vi "test_CCDOpenAndClose.vi"(7 "Test should pass":bool=TRUE, 8 "error in":errorcluster, 9 "tear down connection":bool=TRUE, 10 "set-up a connection":bool=TRUE, 11 "device selection":enum16{"monochromator", "CCD", "SCD"}(ring)=enum."CCD") -> (0 "error out":errorcluster)   [LabVIEW 2023]
uses:
  Classes/CCD/CCD.lvclass
  <vilib>/addons/_JKI Toolkits/Caraya/classes/Assert/Assert Equal Value and Type_Variant.vi
  <vilib>/addons/_JKI Toolkits/Caraya/classes/Assert/Assert Not Error.vi
  <vilib>/addons/_JKI Toolkits/Caraya/classes/Test/Test.lvclass
  <vilib>/addons/_JKI Toolkits/Caraya/classes/Assert/Assert.lvclass
panel:
  # "Connector Pane"
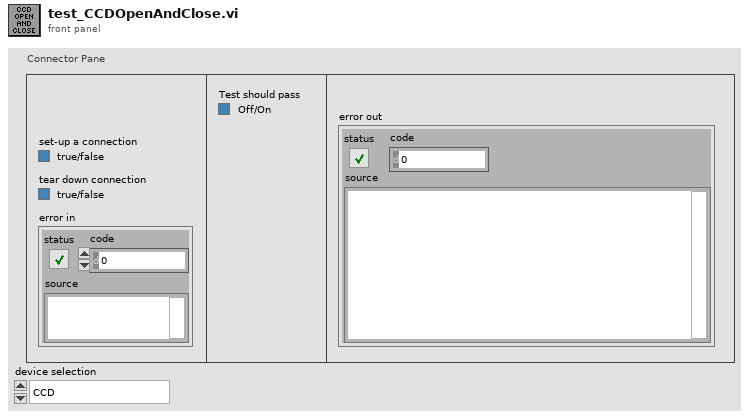
[diagram p1: front panel]
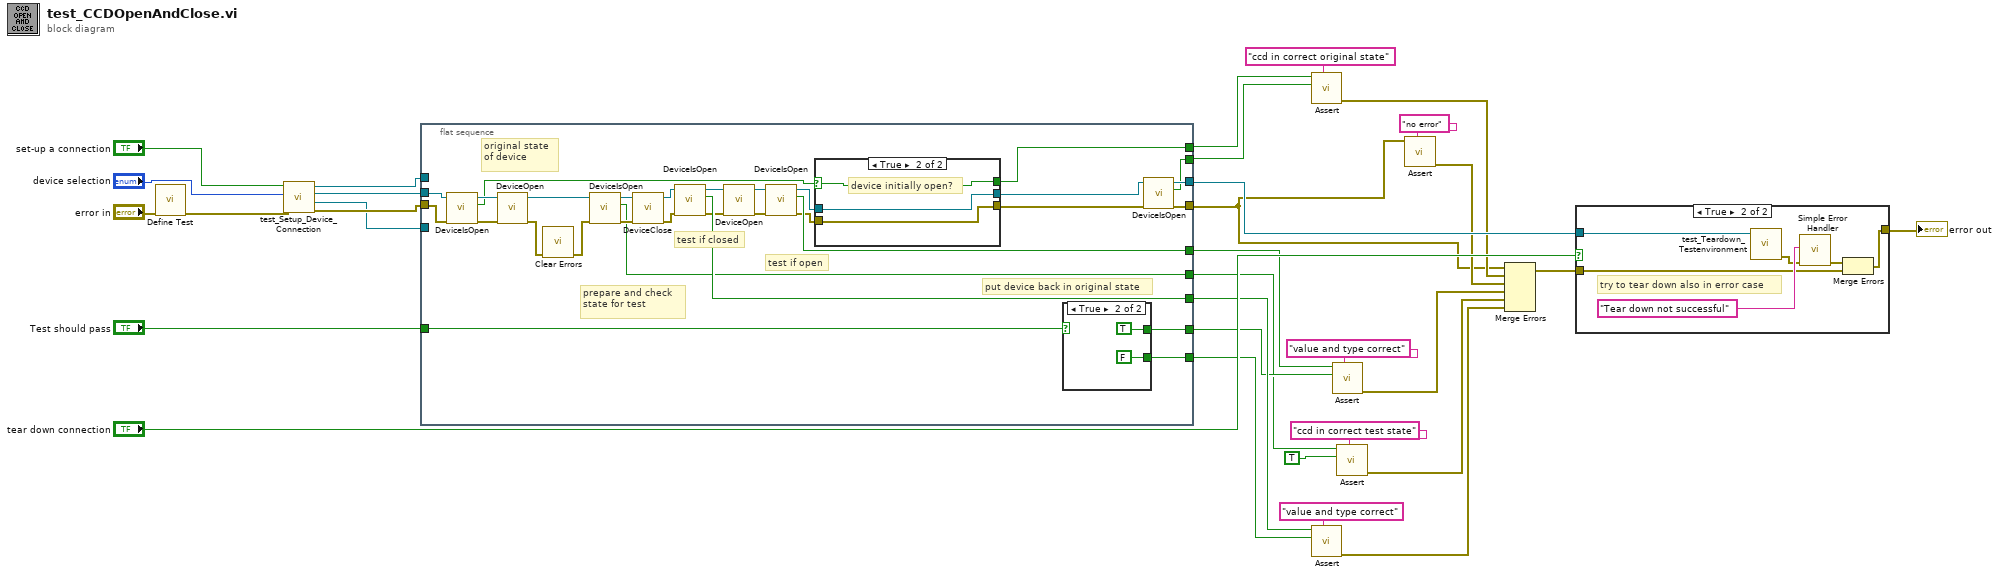
[diagram p0: block diagram]
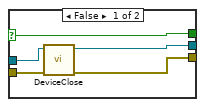
[diagram p2: hidden frame]
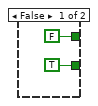
[diagram p3: hidden frame]
diagram:
  n1 = call <vilib>:"Define Test.vi"("error in (no error)"="error in") -> ("error out"=w26:errorcluster)  [unwired: 9 in, 1 out]
  n2 = call "test_Setup_Device_Connection.vi"("error in (no error)"=w26, "device selection"="device selection", "set-up a connection"="set-up a connection") -> ("error out"=w28:errorcluster, "Monochromator out"=w25:refnum<class "Monochromator.lvclass">, "CCD out"=w24:refnum<class "CCD.lvclass">, "SCD out"=w8:refnum<class "SCD.lvclass">)  [unwired: 5 in]
  n3 = flat-sequence {
    tunnel: w28 -> [w61]
    tunnel: w25 -> [_]
    tunnel: w24 -> [w60]
    tunnel: [w36] -> w2
    tunnel: "Test should pass" -> [w62]
    tunnel: [w40] -> w20
    tunnel: [w53] -> w19
    tunnel: [w52] -> w18
    tunnel: [w51] -> w17
    tunnel: [w50] -> w16
    tunnel: [w49] -> w14
    tunnel: [w42] -> w11
    tunnel: [w39] -> w10
    tunnel: w8 -> [_]
    frame #0 {
      # "put device back in original state"
      # "test if open"
      # "test if closed"
      # "original state of device"
      # "prepare and check state for test"
      n4 = call-dynamic "DeviceIsOpen.vi"("error in (no error)"=w61, "CCD in"=w60) -> ("error out"=w35:errorcluster, "device is open?"=w48:bool, "CCD out"=w59:refnum<class "CCD.lvclass">)  [unwired: 6 in, 1 out]
      n5 = call-dynamic "DeviceOpen.vi"("error in (no error)"=w35, "CCD in"=w59) -> ("error out"=w34:errorcluster, "CCD out"=w58:refnum<class "CCD.lvclass">)  [unwired: 6 in, 2 out]
      n6 = call <vilib>:"Clear Errors.vi"("error in (no error)"=w34) -> ("error out"=w33:errorcluster)  [unwired: 5 in, 1 out]
      n7 = call-dynamic "DeviceIsOpen.vi"("error in (no error)"=w33, "CCD in"=w58) -> ("error out"=w54:errorcluster, "device is open?"=w49:bool, "CCD out"=w57:refnum<class "CCD.lvclass">)  [unwired: 6 in, 1 out]
      n8 = call-dynamic "DeviceClose.vi"("error in (no error)"=w54, "CCD in"=w57) -> ("error out"=w55:errorcluster, "CCD out"=w56:refnum<class "CCD.lvclass">)  [unwired: 5 in, 3 out]
      n9 = call-dynamic "DeviceIsOpen.vi"("error in (no error)"=w55, "CCD in"=w56) -> ("error out"=w44:errorcluster, "device is open?"=w53:bool, "CCD out"=w46:refnum<class "CCD.lvclass">)  [unwired: 6 in, 1 out]
      n10 = call-dynamic "DeviceOpen.vi"("error in (no error)"=w44, "CCD in"=w46) -> ("error out"=w43:errorcluster, "CCD out"=w45:refnum<class "CCD.lvclass">)  [unwired: 6 in, 2 out]
      n11 = call-dynamic "DeviceIsOpen.vi"("error in (no error)"=w43, "CCD in"=w45) -> ("error out"=w38:errorcluster, "device is open?"=w51:bool, "CCD out"=w47:refnum<class "CCD.lvclass">)  [unwired: 6 in, 1 out]
      n12 = case shown="True" w48 {
        selector: w48 -> [w65 w68]
        tunnel: w47 -> [w67 w70]
        tunnel: [w66 w70] -> w41
        tunnel: [w65 w68] -> w42
        tunnel: w38 -> [w64 w69]
        tunnel: [w63 w69] -> w37
        frame False {
          n13 = call-dynamic "DeviceClose.vi"("error in (no error)"=w64, "CCD in"=w67) -> ("error out"=w63:errorcluster, "CCD out"=w66:refnum<class "CCD.lvclass">)  [unwired: 5 in, 3 out]
        }
        frame True {
          # "device initially open?"
        }
      }
      n14 = case shown="True" w62 {
        tunnel: [TRUE ("device is open?") FALSE ("device is open?")] -> w52
        tunnel: [FALSE ("device is open?") TRUE ("device is open?")] -> w50
        frame False {
        }
        frame True {
        }
      }
      n15 = call-dynamic "DeviceIsOpen.vi"("error in (no error)"=w37, "CCD in"=w41) -> ("error out"=w36:errorcluster, "device is open?"=w39:bool, "CCD out"=w40:refnum<class "CCD.lvclass">)  [unwired: 6 in, 1 out]
    }
  }
  n16 = call-poly <vilib>:"Assert.vi"("Label"="ccd in correct original state" ("Label (VI Title)"), "Y"=w10, "X"=w11) -> ("error out"=w3:errorcluster)  [unwired: 7 in, 1 out]
  n17 = call-poly <vilib>:"Assert.vi"("Label"="value and type correct" ("Label (VI Title)"), "Y"=w18, "X"=w19) -> ("error out"=w5:errorcluster)  [unwired: 7 in, 1 out]
  n18 = call-poly <vilib>:"Assert.vi"("Label"="value and type correct" ("Label (VI Title)"), "Y"=w16, "X"=w17) -> ("error out"=w30:errorcluster)  [unwired: 7 in, 1 out]
  n19 = call-poly <vilib>:"Assert.vi"("Label"="ccd in correct test state" ("Label (VI Title)"), "Y"=TRUE ("device is open?"), "X"=w14) -> ("error out"=w6:errorcluster)  [unwired: 7 in, 1 out]
  n20 = call-poly <vilib>:"Assert.vi"("Label"="no error" ("Label (VI Title)"), "Not Error?"=w2) -> ("error out"=w4:errorcluster)  [unwired: 8 in, 1 out]
  n21 = Merge Errors(w2, w3, w4, w30, w6, w5) -> (w1:errorcluster)
  n22 = case shown="True" "tear down connection" {
    tunnel: w20 -> [_ w80]
    tunnel: [w75 w76] -> w9
    tunnel: w1 -> [w75 w77]
    frame False {
    }
    frame True {
      # "try to tear down also in error case"
      n23 = call "test_Teardown_Testenvironment.vi"("GenericDevice.lvclass"=w80) -> ("error out"=w79:errorcluster)  [unwired: 9 in, 1 out]
      n24 = call <vilib>:"Simple Error Handler.vi"("error source (\" \")"="Tear down not successful" ("error source (\" \")"), "error in (no error)"=w79) -> ("error out"=w78:errorcluster)  [unwired: 3 in, 4 out]
      n25 = Merge Errors(w78, w77) -> (w76:errorcluster)
    }
  }
  "error out" <- w9
